vi "Update Label.vi"(8 "error in (no error)":errorcluster, 10 "Label in":string, 11 "Rename in":refnum<class "ProjectItem.lvclass">) -> (0 "error out":errorcluster, 1 "New Label?":bool, 2 "Label out":string, 3 "Rename out":refnum<class "ProjectItem.lvclass">)   [LabVIEW 2019, in "ProjectItem.lvclass"]
uses:
  ProjectItem.lvclass
  ProjectItem.lvclass/ProjectItem.ctl
  <vilib>/regexp/Match Regular Expression.xnode
panel:
  out "whole match":string
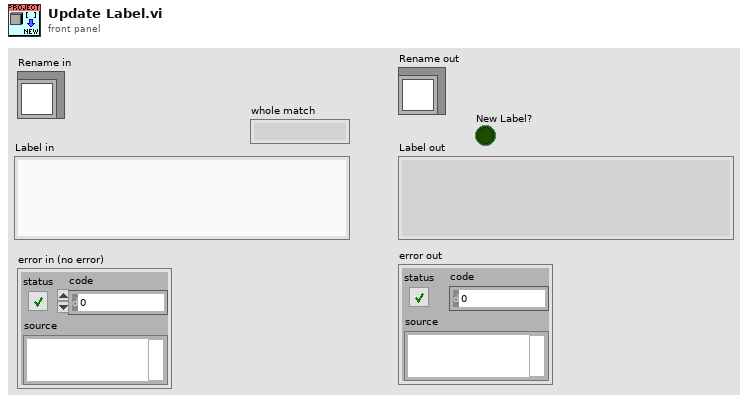
[diagram p1: front panel]
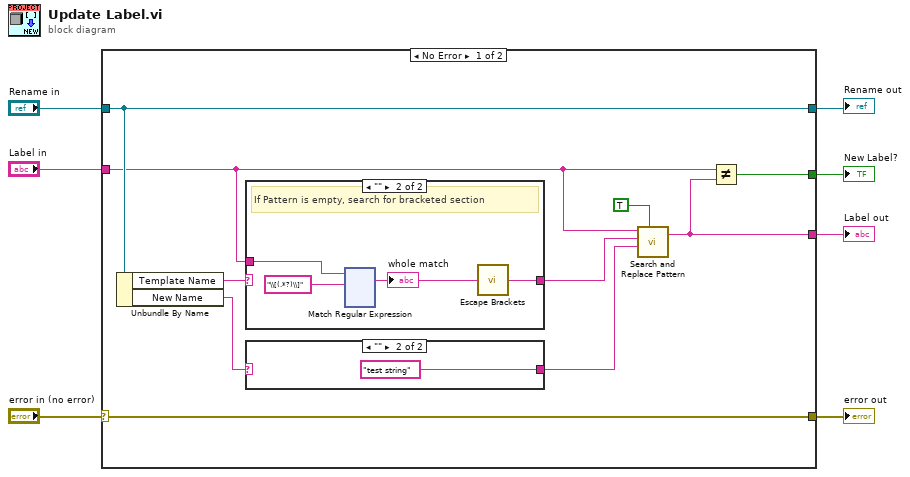
[diagram p0: block diagram]
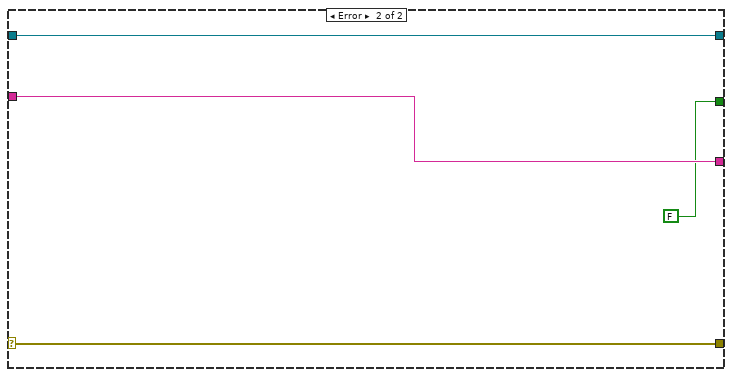
[diagram p4: hidden frame]
diagram:
  n1 = case shown="No Error" "error in (no error)" {
    selector: "error in (no error)" -> [w9 w142]
    tunnel: "Rename in" -> [w17 w141]
    tunnel: [w9 w142] -> w5
    tunnel: [w17 w141] -> w4
    tunnel: [w15 FALSE] -> w2
    tunnel: [w10 w140] -> w3
    tunnel: "Label in" -> [w8 w140]
    frame No Error {
      n2 = Unbundle By Name(w17) -> ("Template Name"=w14:string, "New Name"=w11:string)
      n3 = case shown="\"\"" w14 {
        selector: w14 -> [w20 _]
        tunnel: w8 -> [_ w21]
        tunnel: [w20 w22] -> w13
        frame Default {
        }
        frame "" {
          # "If Pattern is empty, search for bracketed section"
          n4 = xnode "Match Regular Expression"("input string"=w21, "regular expression"="\\[(.*?)\\]") -> ("whole match"=w23:string)  [unwired: 4 in, 4 out]
          "whole match" <- w23
          n5 = call "Escape Brackets.vi"("Pattern"=w23) -> ("result string"=w22:string)
        }
      }
      n6 = case shown="\"\"" w11 {
        selector: w11 -> [w18 _]
        tunnel: [w18 "test string"] -> w12
        frame Default {
        }
        frame "" {
        }
      }
      n7 = call <vilib>:"Search and Replace Pattern.vi"("string"=w8, "regular expression (\"\")"=w13, "replace string (\"\")"=w12, "replace all? (F)"=TRUE) -> ("result string"=w10:string)  [unwired: 1 in, 1 out]
      n8 = Not Equal?(x=w8, y=w10) -> (x != y?=w15:bool)
    }
    frame Error {
    }
  }
  "Rename out" <- w4
  "error out" <- w5
  "Label out" <- w3
  "New Label?" <- w2
